vi "Produce Pattern TEST.vi"() -> ()   [LabVIEW 2016]
uses:
  <vilib>/Utility/sysdir.llb/System Directory Type.ctl
panel:
  out "standard error":string
  out "standard output":string
  out "error out":errorcluster
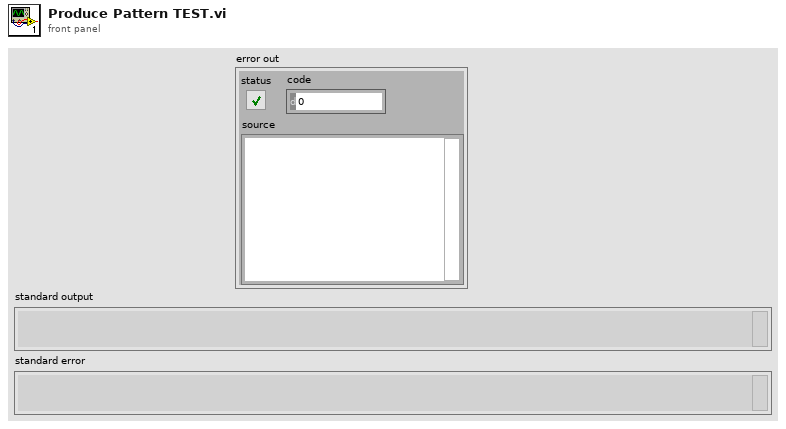
[diagram p1: front panel]
types:
  T1 = typedef "System Directory Type.ctl" = i32
  T2 = enum16{"open", "replace", "create", "open or create", "replace or create", "replace or create with confirmation"}
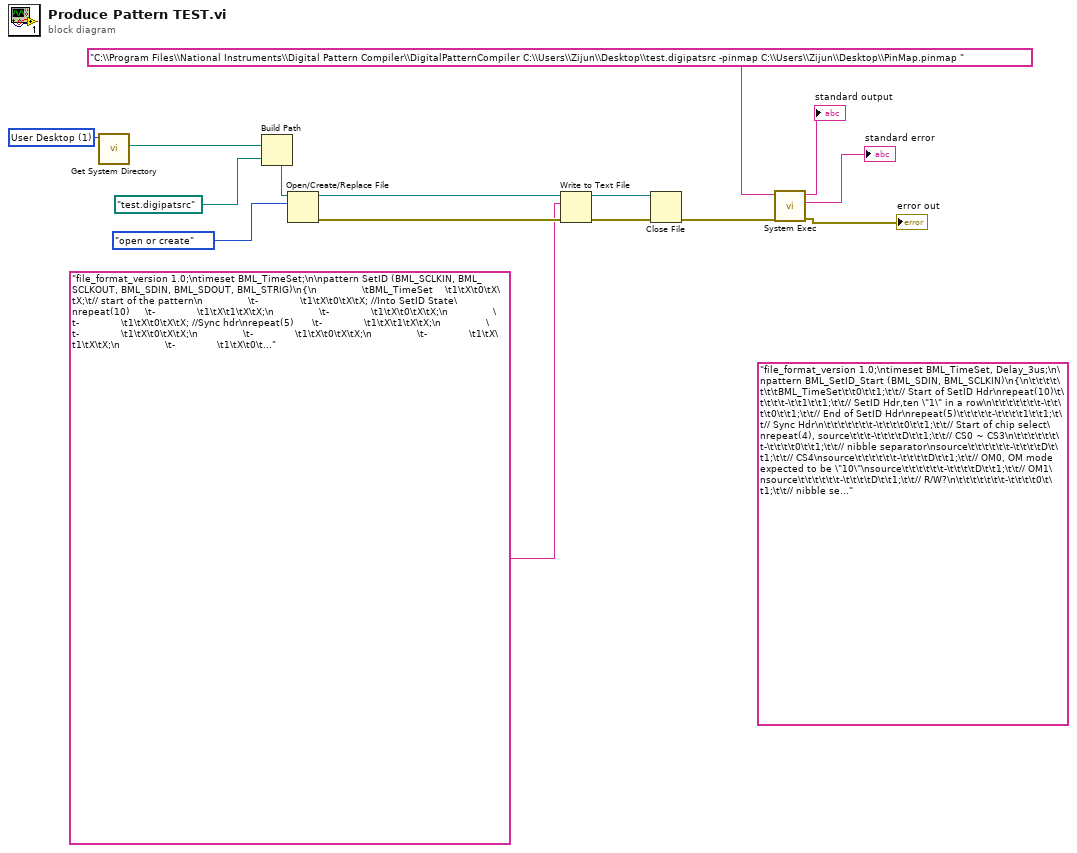
[diagram p0: block diagram]
diagram:
  w10 = T1 1 items=["User Home"=0, "User Desktop"=1, "User Documents"=2, "User Application Data"=3, "User Preferences"=4, "User Temporary"=5, "Public Documents"=6, "Public Application Data"=7, "Public Preferences"=8, "Public Cache"=13, "System Core Libraries"=9, "System Installed Libraries"=10, "Application Files"=11, "Boot Volume Root"=12] ("system directory type")
  (unwired) "file_format_version 1.0;\ntimeset BML_TimeSet, Delay_3us;\n\npattern BML_SetID_Start (BML_SDIN, BML_SCLKIN)\n{\n\t\t\t\t\t\t\tBML_TimeSet\t\t0\t\t1;\t\t// Start of SetID Hdr\nrepeat(10)\t\t\t\t\t-\t\t1\t\t1;\t\t// SetID Hdr,ten \"1\" in a row\n\t\t\t\t\t\t\t-\t\t\t\t0\t\t1;\t\t// End of SetID Hdr\nrepeat(5)\t\t\t\t\t-\t\t\t\t1\t\t1;\t\t// Sync Hdr\n\t\t\t\t\t\t\t-\t\t\t\t0\t\t1;\t\t// Start of chip select\nrepeat(4), source\t\t\t-\t\t\t\tD\t\t1;\t\t// CS0 ~ CS3\n\t\t\t\t\t\t\t-\t\t\t\t0\t\t1;\t\t// nibble separator\nsource\t\t\t\t\t\t-\t\t\t\tD\t\t1;\t\t// CS4\nsource\t\t\t\t\t\t-\t\t\t\tD\t\t1;\t\t// OM0, OM mode expected to be \"10\"\nsource\t\t\t\t\t\t-\t\t\t\tD\t\t1;\t\t// OM1\nsource\t\t\t\t\t\t-\t\t\t\tD\t\t1;\t\t// R/W?\n\t\t\t\t\t\t\t-\t\t\t\t0\t\t1;\t\t// nibble separator\nrepeat(4), source\t\t\t-\t\t\t\tD\t\t1;\t\t// BL0 ~ BL3\n\t\t\t\t\t\t\t-\t\t\t\t0\t\t1;\t\t// nibble separator\nrepeat(4), source\t\t\t-\t\t\t\tD\t\t1;\t\t// FSN0 ~ FSN3\n\t\t\t\t\t\t\t-\t\t\t\t0\t\t1;\t\t// nibble separator\nhalt\t\t\t\t\t\t-\t\t\t\tX\t\tX;\n}\n"
  n1 = call <vilib>:"Get System Directory.vi"("system directory type"=w10) -> ("system directory"=w9:path)  [unwired: 10 in]
  n2 = Build Path(base path=w9, name or relative path=path "test.digipatsrc" ("file path (use dialog)")) -> (appended path=w7:path)
  n3 = Open/Create/Replace File(file path (use dialog)=w7, operation (0:open)=T2."open or create") -> (refnum out=w14:refnum<file>, error out=w13:errorcluster)  [unwired: 4 in, 1 out]
  n4 = Write to Text File(file (use dialog)=w14, text="file_format_version 1.0;\ntimeset BML_TimeSet;\n\npattern SetID (BML_SCLKIN, BML_SCLKOUT, BML_SDIN, BML_SDOUT, BML_STRIG)\n{\n               \tBML_TimeSet    \t1\tX\t0\tX\tX;\t// start of the pattern\n               \t-              \t1\tX\t0\tX\tX; //Into SetID State\nrepeat(10)     \t-              \t1\tX\t1\tX\tX;\n               \t-              \t1\tX\t0\tX\tX;\n               \t-              \t1\tX\t0\tX\tX; //Sync hdr\nrepeat(5)      \t-              \t1\tX\t1\tX\tX;\n               \t-              \t1\tX\t0\tX\tX;\n               \t-              \t1\tX\t0\tX\tX;\n               \t-              \t1\tX\t1\tX\tX;\n               \t-              \t1\tX\t0\tX\tX;\n               \t-              \t1\tX\t0\tX\tX;\n               \t-              \t1\tX\t0\tX\tX;\n               \t-              \t1\tX\t0\tX\tX;\n               \t-              \t1\tX\t0\tX\tX;\n               \t-              \t1\tX\t0\tX\tX;\n               \t-              \t1\tX\t1\tX\tX;\n               \t-              \t1\tX\t0\tX\tX;\n               \t-              \t1\tX\t0\tX\tX;\n               \t-              \t1\tX\t0\tX\tX;\n               \t-              \t1\tX\t0\tX\tX;\n               \t-              \t1\tX\t0\tX\tX;\n               \t-              \t1\tX\t0\tX\tX;\n               \t-              \t1\tX\t0\tX\tX;\n               \t-              \t1\tX\t0\tX\tX;\n               \t-              \t1\tX\t0\tX\tX;\n               \t-              \t1\tX\t0\tX\tX;\n               \t-              \t1\tX\t0\tX\tX;\nrepeat(50)     \t-              \t1\tX\t0\tX\tX; //Wait for 50 Timeset\nrepeat(10)     \t-              \t1\tX\t0\tX\tX; //out SetID state\nrepeat(15)     \t-              \t1\tX\t1\tX\tX;\nrepeat(10)     \t-              \t1\tX\t0\tX\tX;\nhalt           \t-              \tX\tX\tX\tX\tX;\n}", error in=w13) -> (refnum out=w12:refnum<file>, error out=w11:errorcluster)  [unwired: 1 in, 1 out]
  n5 = Close File(refnum=w12, error in=w11) -> (error out=w6:errorcluster)  [unwired: 1 out]
  n6 = call <vilib>:"System Exec.vi"("error in (no error)"=w6, "command line"="C:\\Program Files\\National Instruments\\Digital Pattern Compiler\\DigitalPatternCompiler C:\\Users\\Zijun\\Desktop\\test.digipatsrc -pinmap C:\\Users\\Zijun\\Desktop\\PinMap.pinmap ") -> ("error out"=→"error out":errorcluster, "standard error"=→"standard error":string, "standard output"=→"standard output":string)  [unwired: 6 in, 1 out]
